vi "FGV_WriteFetchDataToListboxandGraph.vi"(7 "Mode":T1, 8 "error in (no error)":errorcluster, 10 "FetchDataString":string="0.1, 1.5, 1, 10.5, 10, 0.2, 2.5, 2, 20.5, 20, 0.3, 3.5, 3, 30.5, 30", 11 "Common Refs":T2={"LBox_ChList"=refnum, "STR_LoggingChName1"=refnum, "Listbox_ChValue"=refnum, "STR_LoggingChName2"=refnum, "STR_LoggingChName3"=refnum, "STR_LoggingChName4"=refnum, "STR_LoggingChName5"=refnum, "STR_LoggingChName6"=refnum, "OXY_SCPI Ref"="TCPIP0::192.168.1.75::10001::SOCKET", "STR_ChName1"=refnum, "STR_ChName2"=refnum, "STR_ChName3"=refnum, "STR_ChName4"=refnum, "STR_ChName5"=refnum, "STR_ChName6"=refnum, "Enum_SelectTimestampFormat"=refnum, "GRAPH-XY_ELOG"=refnum, "GRAPH-XY_Measurement"=refnum, "Button_StartBuffer"=refnum, "Button_StopBuffer"=refnum, "Button_FetchData"=refnum, "STR_LoggingChName1"=refnum, "STR_LoggingChName2"=refnum, "STR_LoggingChName3"=refnum, "STR_LoggingChName4"=refnum, "STR_LoggingChName5"=refnum, "STR_LoggingChName6"=refnum, "Enum_SelectCalc"=refnum, "Num_SetDurationTime"=refnum, "Button_StopTransfer"=refnum, "Button_StartTransfer"=refnum, "STR_IN_AggregationRate"=refnum, "Button_Disconnect"=refnum, "Button_Connect"=refnum, "Button_StartRec"=refnum, "Button_PauseRec"=refnum, "Button_StopRec"=refnum, "Bool_StatusLED"=refnum, "Indicator_RecordingStatus"=refnum}) -> (0 "error out":errorcluster)   [LabVIEW 2018]
uses:
  TypeDefs/Refs_Common.ctl
  TypeDefs/TD_Case_ELOG-ManageGUI.ctl
  TypeDefs/Graph_DataArrayElement.ctl
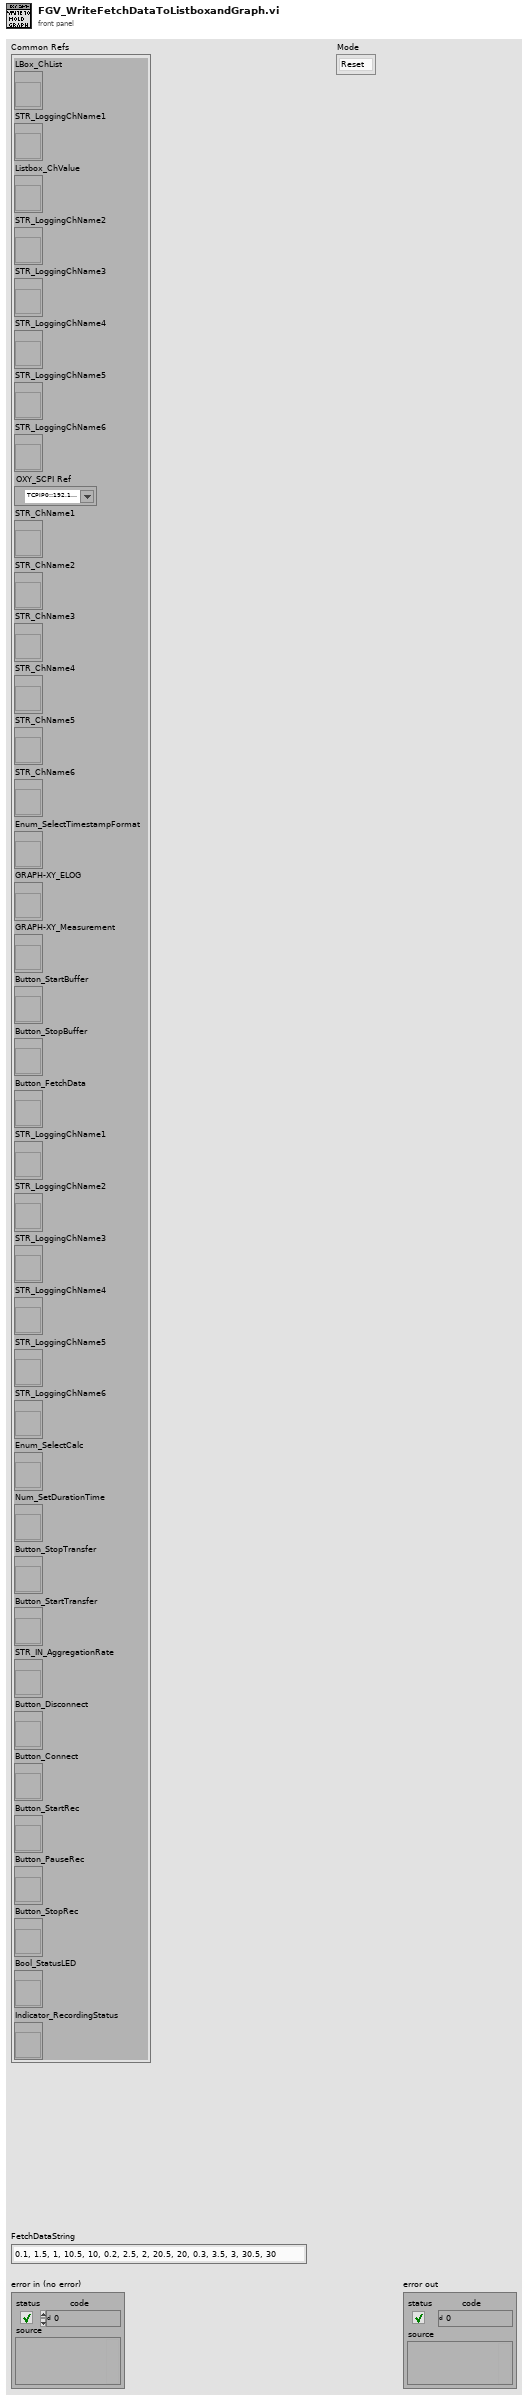
[diagram p1: front panel]
types:
  T1 = typedef "TD_Case_ELOG-ManageGUI.ctl" = enum16{"Reset", "AddDataToGUI"}
  T2 = typedef "Refs_Common.ctl" = cluster{"LBox_ChList":refnum<vi>, "STR_LoggingChName1":refnum<vi>, "Listbox_ChValue":refnum<vi>, "STR_LoggingChName2":refnum<vi>, "STR_LoggingChName3":refnum<vi>, "STR_LoggingChName4":refnum<vi>, "STR_LoggingChName5":refnum<vi>, "STR_LoggingChName6":refnum<vi>, "OXY_SCPI Ref":refnum<visa-resource-name>, "STR_ChName1":refnum<vi>, "STR_ChName2":refnum<vi>, "STR_ChName3":refnum<vi>, "STR_ChName4":refnum<vi>, "STR_ChName5":refnum<vi>, "STR_ChName6":refnum<vi>, "Enum_SelectTimestampFormat":refnum<vi>, "GRAPH-XY_ELOG":refnum<vi>, "GRAPH-XY_Measurement":refnum<vi>, "Button_StartBuffer":refnum<vi>, "Button_StopBuffer":refnum<vi>, "Button_FetchData":refnum<vi>, "STR_LoggingChName1":refnum<vi>, "STR_LoggingChName2":refnum<vi>, "STR_LoggingChName3":refnum<vi>, "STR_LoggingChName4":refnum<vi>, "STR_LoggingChName5":refnum<vi>, "STR_LoggingChName6":refnum<vi>, "Enum_SelectCalc":refnum<vi>, "Num_SetDurationTime":refnum<vi>, "Button_StopTransfer":refnum<vi>, "Button_StartTransfer":refnum<vi>, "STR_IN_AggregationRate":refnum<vi>, "Button_Disconnect":refnum<vi>, "Button_Connect":refnum<vi>, "Button_StartRec":refnum<vi>, "Button_PauseRec":refnum<vi>, "Button_StopRec":refnum<vi>, "Bool_StatusLED":refnum<vi>, "Indicator_RecordingStatus":refnum<vi>}
  T3 = cluster{"Timestamp":timestamp[], "Value":dbl[]}[]
  T4 = typedef "Graph_DataArrayElement.ctl" = cluster{"Timestamp":timestamp[], "Value":dbl[]}
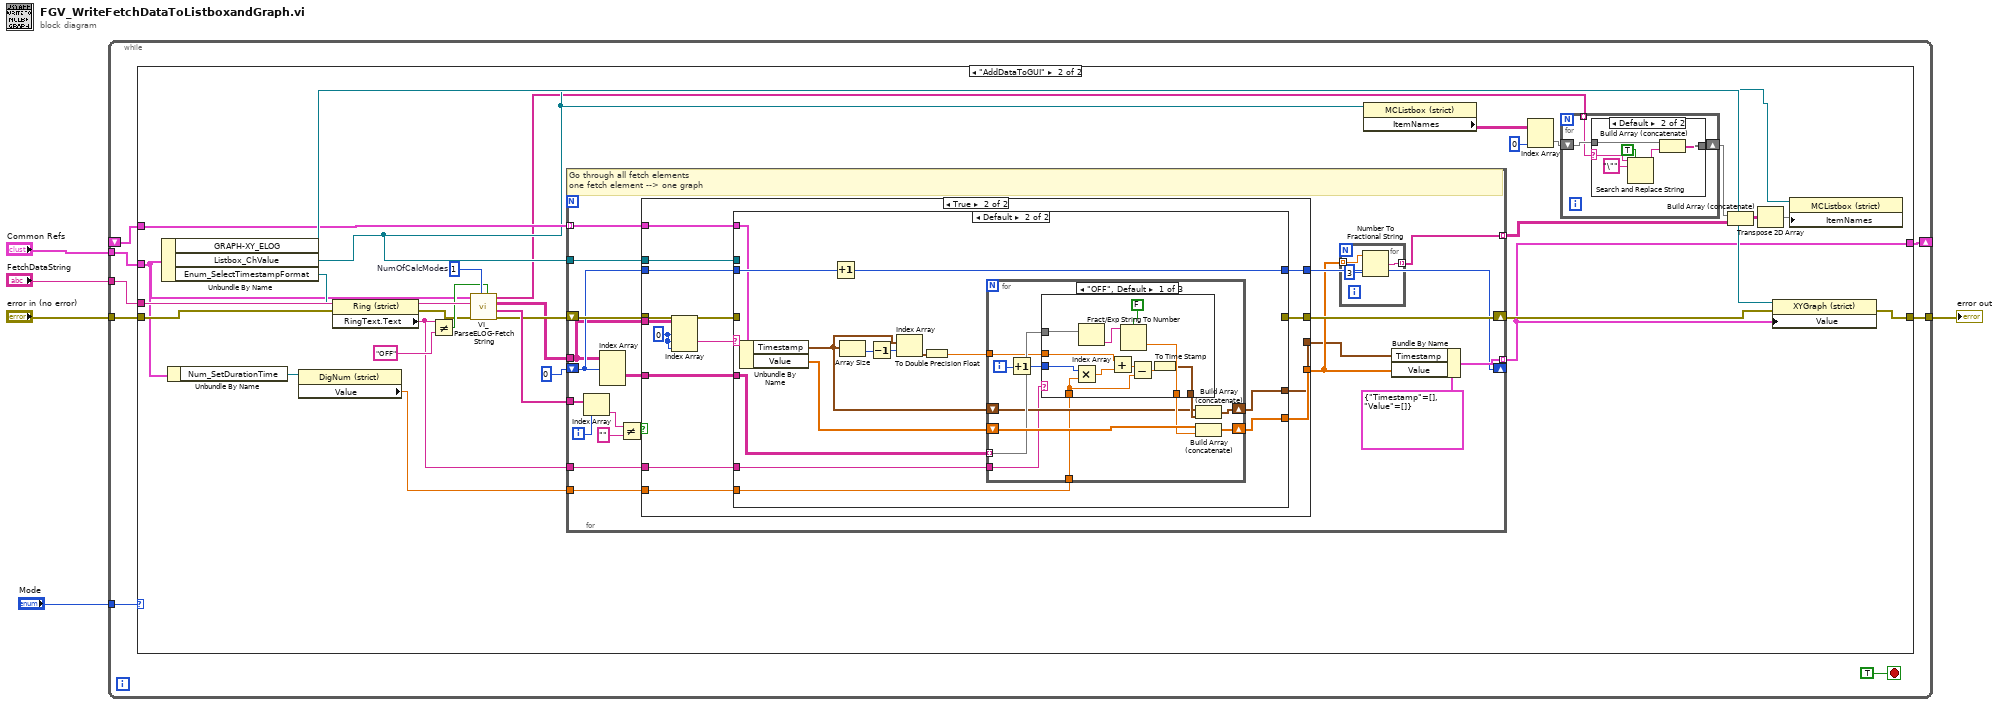
[diagram p0: block diagram]
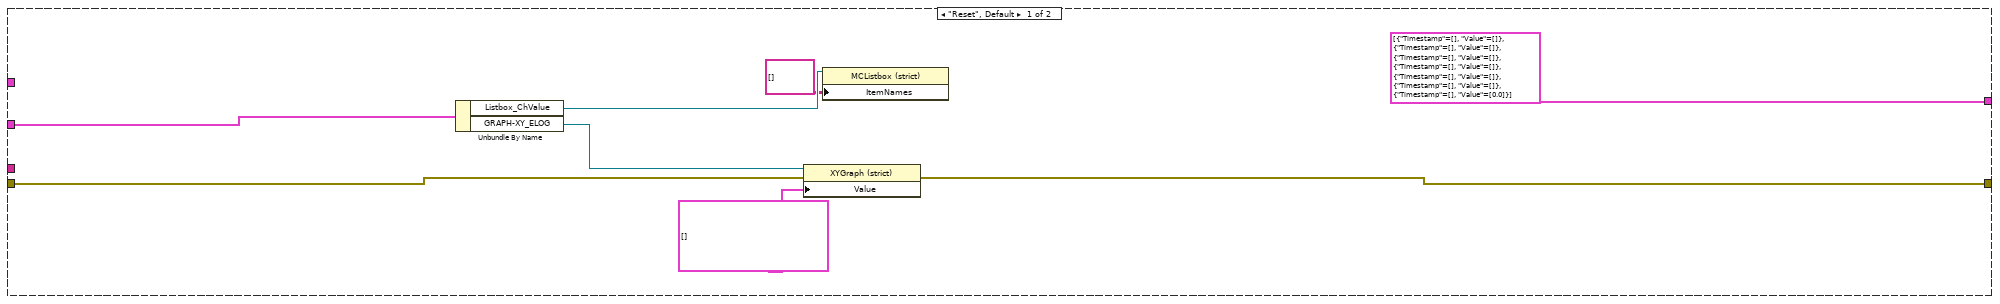
[diagram p2: hidden frame]
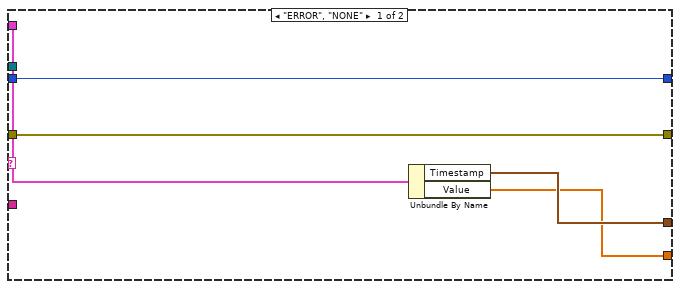
[diagram p5: hidden frame]
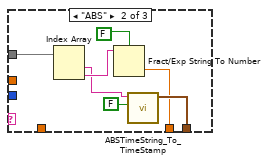
[diagram p6: hidden frame]
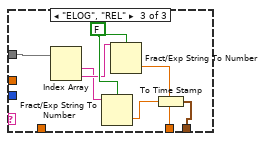
[diagram p7: hidden frame]
diagram:
  n1 = while {
    tunnel: "error in (no error)" -> [w13]
    tunnel: "FetchDataString" -> [w12]
    tunnel: "Common Refs" -> [w11]
    tunnel: "Mode" -> [w10]
    shift-right: [w7] -> _
    shift-left: _ -> [w8]
    tunnel: [w6] -> w1
    stop <- TRUE stop-if-true
    n2 = case shown="\"AddDataToGUI\"" w10 {
      tunnel: w13 -> [w18 w35]
      tunnel: w12 -> [_ w50]
      tunnel: w11 -> [w19 w23]
      tunnel: w8 -> [_ w46]
      tunnel: [T4[] [{"Timestamp"=[], "Value"=[]}, {"Timestamp"=[], "Value"=[]}, {"Timestamp"=[], "Value"=[]}, {"Timestamp"=[], "Value"=[]}, {"Timestamp"=[], "Value"=[]}, {"Timestamp"=[], "Value"=[]}, {"Timestamp"=[], "Value"=[0.0]}] w33] -> w7
      tunnel: [w17 w44] -> w6
      frame "Reset", Default {
        n3 = Unbundle By Name(w19) -> ("Listbox_ChValue"=w15:refnum<vi>, "GRAPH-XY_ELOG"=w20:refnum<vi>)
        n4 = property class="XYGraph (strict)"(reference=w20, error in=w18, "Value"=T3 []) -> (error out=w17:errorcluster)  [unwired: 1 out]
        n5 = property class="MCListbox (strict)"(reference=w15, "ItemNames"=string[][] [] ("Item Names")) -> ()  [unwired: 1 in, 2 out]
      }
      frame "AddDataToGUI" {
        w48 = 1  # NumOfCalcModes
        n6 = Unbundle By Name(w23) -> ("GRAPH-XY_ELOG"=w47:refnum<vi>, "Listbox_ChValue"=w30:refnum<vi>, "Enum_SelectTimestampFormat"=w40:refnum<vi>)
        n7 = Unbundle By Name(w23) -> ("Num_SetDurationTime"=w24:refnum<vi>)
        n8 = property class="DigNum (strict)"(reference=w24) -> ("Value"=w22:dbl)  [unwired: 1 in, 2 out]
        n9 = property class="Ring (strict)"(reference=w40, error in=w35) -> (error out=w36:errorcluster, "RingText.Text"=w38:string)  [unwired: 1 out]
        n10 = Not Equal?(x=w38, y="OFF") -> (x != y?=w37:bool)
        n11 = call "VI_ParseELOG-FetchString.vi"("TimestampIncluded"=w37, "NumOfCalcModes"=w48, "error in (no error)"=w36, "FetchDataString"=w50, "Common Refs"=w23) -> ("error out"=w43:errorcluster, "Corrected_LoggingChName"=w49:string[], "Fomarted List"=w42:string[][][], "Timestamp only list"=w26:string[])  [unwired: 3 in]
        n12 = for {
          tunnel: w49 -> [w80]
          tunnel: w30 -> [w66]
          tunnel: w42 -> [w68]
          tunnel: w46 -> [w69] mode=indexing
          tunnel: [w74] -> w33 mode=indexing
          shift-right: [w73] -> w45
          shift-left: w43 -> [w72]
          shift-right: [w70] -> _
          shift-left: 0 -> [w71]
          tunnel: w38 -> [w64]
          tunnel: [w62] -> w34 mode=indexing
          tunnel: w22 -> [w61]
          i -> [w67]
          # "Go through all fetch elements\none fetch element --> one graph"
          n13 = Index Array(array=w80, index=w67) -> (element=w79:string)
          n14 = Index Array(array=w68, index (dim 0)=w71) -> (element=w77:string[][])  [unwired: 2 in]
          n15 = Not Equal?(x=w79, y="") -> (x != y?=w76:bool)
          n16 = case shown="True" w76 {
            tunnel: w66 -> [_ w96]
            tunnel: w77 -> [_ w92]
            tunnel: [w82 w85] -> w73
            tunnel: w72 -> [w82 w95]
            tunnel: w71 -> [w81 w94]
            tunnel: [w81 w93] -> w70
            tunnel: [_ w91] -> w65
            tunnel: [_ w90] -> w63
            tunnel: w69 -> [_ w89]
            tunnel: w68 -> [_ w88]
            tunnel: w64 -> [_ w84]
            tunnel: w61 -> [_ w83]
            frame False {
            }
            frame True {
              w87 = 0 ("index (page)")
              n17 = Index Array(array=w88, index (dim 0)=w87, index (dim 1)=w87, index (dim 2)=w87) -> (element=w86:string)
              n18 = case shown="Default" w86 {
                tunnel: w96 -> [_ _]
                tunnel: [w98 _] -> w85
                tunnel: w95 -> [w98 _]
                tunnel: w94 -> [w97 w115]
                tunnel: [w97 w114] -> w93
                tunnel: w92 -> [_ w103]
                tunnel: [w99 w113] -> w91
                tunnel: [w100 w112] -> w90
                tunnel: w89 -> [w101 w110]
                tunnel: w84 -> [_ w104]
                tunnel: w83 -> [_ w102]
                frame "ERROR", "NONE" {
                  n19 = Unbundle By Name(w101) -> ("Timestamp"=w100:timestamp[], "Value"=w99:dbl[])
                }
                frame Default {
                  n20 = Unbundle By Name(w110) -> ("Timestamp"=w109:timestamp[], "Value"=w111:dbl[])
                  n21 = Increment(x=w115) -> (x+1=w114:i32)
                  n22 = Array Size(array=w109) -> (size(s)=w108:i32)
                  n23 = Decrement(x=w108) -> (x-1=w107:i32)
                  n24 = Index Array(array=w109, index=w107) -> (element=w106:timestamp)
                  n25 = To Double Precision Float(number=w106) -> (double precision float=w105:dbl)
                  n26 = for {
                    tunnel: w103 -> [w123] mode=indexing
                    shift-right: [w126] -> w112
                    shift-left: w109 -> [w121]
                    shift-right: [w127] -> w113
                    shift-left: w111 -> [w125]
                    tunnel: w105 -> [w120]
                    tunnel: w104 -> [w119]
                    tunnel: w102 -> [w118]
                    i -> [w117]
                    n27 = Increment(x=w117) -> (x+1=w116:i32)
                    n28 = case shown="\"OFF\", Default" w119 {
                      tunnel: [w134 w144 w151] -> w124
                      tunnel: w123 -> [w138 w142 w150]
                      tunnel: [w137 w141 w149] -> w122
                      tunnel: w120 -> [w135 _ _]
                      tunnel: w118 -> [w129 _ _]
                      tunnel: w116 -> [w132 _ _]
                      frame "OFF", Default {
                        n29 = Multiply(x=w132, y=w129) -> (x*y=w131:dbl)
                        n30 = Index Array(array=w138) -> (element=w133:string)  [unwired: 1 in]
                        n31 = Add(x=w135, y=w131) -> (x+y=w130:dbl)
                        n32 = Fract/Exp String To Number(use system decimal point (T)=FALSE, string=w133) -> (number=w137:dbl)  [unwired: 2 in, 1 out]
                        n33 = Subtract(x=w130, y=w129) -> (x-y=w128:dbl)
                        n34 = To Time Stamp(1:w128) -> (0:w134:timestamp)
                      }
                      frame "ABS" {
                        n35 = Index Array(array=w142) -> (element #1=w139:string, element #2=w140:string)  [unwired: 2 in]
                        n36 = Fract/Exp String To Number(use system decimal point (T)=FALSE, string=w140) -> (number=w141:dbl)  [unwired: 2 in, 1 out]
                        n37 = call "ABSTimeString_To_TimeStamp.vi"("is UTC (F)"=FALSE, "Time String"=w139) -> ("Time Stamp"=w144:timestamp)  [unwired: 8 in, 1 out]
                      }
                      frame "ELOG", "REL" {
                        w148 = FALSE ("use system decimal point (T)")
                        n38 = Index Array(array=w150) -> (element #1=w146:string, element #2=w147:string)  [unwired: 2 in]
                        n39 = Fract/Exp String To Number(use system decimal point (T)=w148, string=w146) -> (number=w152:dbl)  [unwired: 2 in, 1 out]
                        n40 = Fract/Exp String To Number(use system decimal point (T)=w148, string=w147) -> (number=w149:dbl)  [unwired: 2 in, 1 out]
                        n41 = To Time Stamp(1:w152) -> (0:w151:timestamp)
                      }
                    }
                    n42 = Build Array (concatenate)(w121, w124) -> (w126:timestamp[])
                    n43 = Build Array (concatenate)(w125, w122) -> (w127:dbl[])
                  }
                }
              }
            }
          }
          n44 = for {
            tunnel: w65 -> [w155] mode=indexing
            tunnel: [w154] -> w62 mode=indexing
            n45 = Number To Fractional String(number=w155, precision (6)=i16 3) -> (F-format string=w154:string)  [unwired: 2 in]
          }
          n46 = Bundle By Name(cluster=T4 {"Timestamp"=[], "Value"=[]} ("Data Element"), "Timestamp"=w63, "Value"=w65) -> (w74:T4)
        }
        n47 = property class="MCListbox (strict)"(reference=w30) -> ("ItemNames"=w29:string[][])  [unwired: 1 in, 2 out]
        n48 = Index Array(array=w29, index (col)=0 ("disabled index (col)")) -> (element=w27:string[])  [unwired: 1 in]
        n49 = for {
          tunnel: w26 -> [w51] mode=indexing
          shift-right: [w52] -> w25
          shift-left: w27 -> [w53]
          n50 = case shown="Default" w51 {
            selector: w51 -> [_ w58]
            tunnel: w53 -> [w54 w60]
            tunnel: [w54 w59] -> w52
            frame "NONE" {
            }
            frame Default {
              n51 = Search and Replace String(replace all?=TRUE ("replace all? (F)"), input string=w58, search string="\"") -> (result string=w55:string)  [unwired: 5 in, 3 out]
              n52 = Build Array (concatenate)(w60, w55) -> (w59:string[])
            }
          }
        }
        n53 = Build Array (concatenate)(w25, w34) -> (w31:string[][])
        n54 = Transpose 2D Array(2D array=w31) -> (transposed array=w32:string[][])
        n55 = property class="XYGraph (strict)"(reference=w47, error in=w45, "Value"=w33) -> (error out=w44:errorcluster)  [unwired: 1 out]
        n56 = property class="MCListbox (strict)"(reference=w30, "ItemNames"=w32) -> ()  [unwired: 1 in, 2 out]
      }
    }
  }
  "error out" <- w1
